vi "PHSensor Event Example.vi"() -> ()   [LabVIEW 2012, in "Phidget PH Sensor.lvlib"]
uses:
  <instrlib>/Phidgets/Phidget PH Sensor/Phidget PH Sensor.lvlib
  <instrlib>/Phidgets/Phidget PH Sensor/Public/PHSensorStart.vi
  <instrlib>/Phidgets/Phidget PH Sensor/Public/PHSensorClose.vi
  <instrlib>/Phidgets/Phidget Common/Phidget Common.lvlib
panel:
  out "pH":dbl format="%.2f"
  in  "stop":bool
  out "Serial Number Return":i32
  in  "Device Info":T1={"Serial Number"=-1, "Channel"=0, "Port"=0}
  out "error out":errorcluster
  # "Be sure to use this stop button to stop the program.\nIf you use the \"Abort Execution\" button, you will\nneed to use PhidgetResetLibrary.vi or restart Labview \nin order for any Phidgets to work."
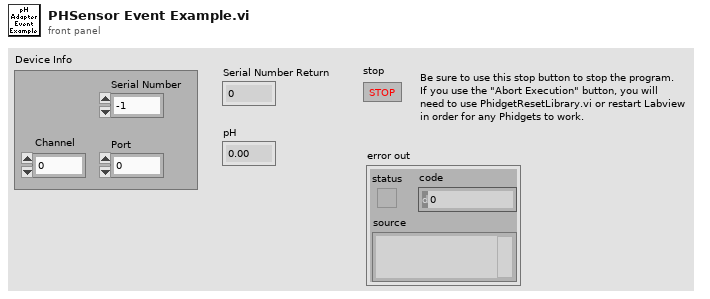
[diagram p1: front panel]
types:
  T1 = cluster{"Serial Number":i32, "Channel":i32, "Port":i32}
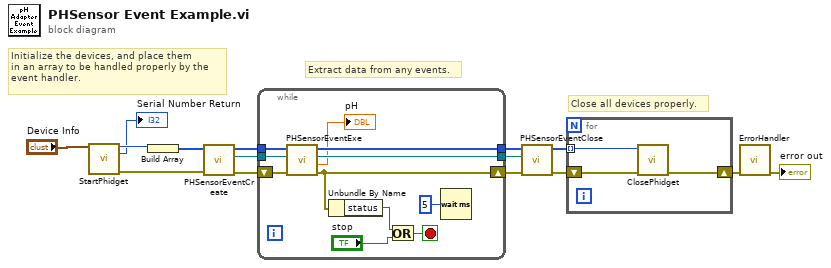
[diagram p0: block diagram]
diagram:
  # "Close all devices properly."
  # "Extract data from any events."
  # "Initialize the devices, and place them\nin an array to be handled properly by the\nevent handler."
  n1 = call-poly <instrlib>:"StartPhidget.vi"("Device Info"="Device Info") -> ("Phidget ID"=w5:u64, "Serial Number Return"=→"Serial Number Return":i32, "error out"=w2:errorcluster)  [unwired: 11 in, 1 out]
  n2 = Build Array(w5) -> (w15:u64[])
  n3 = call <instrlib>:"PHSensorEventCreate.vi"("error in (no error)"=w2, "Devices In"=w15) -> ("error out"=w8:errorcluster, "Event Registration Refnum"=w13:refnum<event-registration>, "Devices Out"=w14:u64[])  [unwired: 7 in]
  n4 = while {
    tunnel: w14 -> [w26]
    tunnel: w13 -> [w21]
    tunnel: [w25] -> w10
    shift-right: [w20] -> w9
    shift-left: w8 -> [w24]
    tunnel: [w22] -> w3
    stop <- w19 stop-if-true
    n5 = call <instrlib>:"PHSensorEventExe.vi"("error in (no error)"=w24, "Event Registration Refnum In"=w21, "Devices In"=w26) -> ("error out"=w20:errorcluster, "pH"=→"pH":dbl, "Event Registration Refnum Out"=w25:refnum<event-registration>, "Devices Out"=w22:u64[])  [unwired: 2 in, 3 out]
    n6 = Unbundle By Name(w20) -> ("status"=w17:bool)
    n7 = Or(x=w17, y="stop") -> (x .or. y?=w19:bool)
    n8 = Wait (ms)(milliseconds to wait=u32 5) -> ()  [unwired: 1 out]
  }
  n9 = call <instrlib>:"PHSensorEventClose.vi"("error in (no error)"=w9, "Event Registration Refnum In"=w10, "Devices In"=w3) -> ("error out"=w6:errorcluster, "Devices Out"=w4:u64[])  [unwired: 7 in]
  n10 = for {
    tunnel: w4 -> [w27] mode=indexing
    shift-right: [w29] -> w12
    shift-left: w6 -> [w28]
    n11 = call-poly <instrlib>:"ClosePhidget.vi"("error in"=w28, "Device In"=w27) -> ("error out"=w29:errorcluster)  [unwired: 9 in]
  }
  n12 = call <instrlib>:"ErrorHandler.vi"("error in"=w12) -> ("error out"=→"error out":errorcluster)  [unwired: 9 in, 1 out]
